vi "wykonajRuch.vi"(8 "error in (no error)":errorcluster, 9 "Wybór komory":T1, 10 "Akcja":T2=enum."Sprawdź", 11 "LINX Resource in":T3) -> (0 "error out":errorcluster, 3 "LINX Resource out":T3)   [LabVIEW 2014]
uses:
  <vilib>/MakerHub/LINX/Private/Type Defs/LINX Ref.ctl
  <vilib>/MakerHub/LINX/Private/Type Defs/Platform.ctl
  <vilib>/MakerHub/LINX/Private/Type Defs/Interface.ctl
  <vilib>/MakerHub/LINX/Private/Device/Type Defs/LINX Device Config.ctl
  <vilib>/MakerHub/LINX/Private/Device/Type Defs/TCP Config.ctl
  <vilib>/MakerHub/LINX/Private/Device/Type Defs/Channels.ctl
  wczytajDaneDoRuchuVIs/Akcje_wczytywania_danych_do_ruchu.ctl
  wykonajRuchVIs/parametryKomorVIs/Wybor_komory.ctl
  Akcja_kontrolki.ctl
  <vilib>/MakerHub/LINX/LMH-LINX.lvlib
  <vilib>/MakerHub/LINX/Private/Device/Device.lvlib
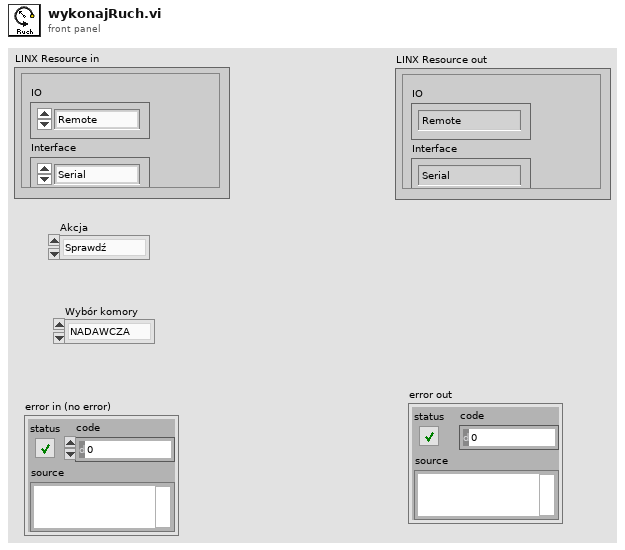
[diagram p1: front panel]
types:
  T1 = typedef "Wybor_komory.ctl" = enum16{"NADAWCZA", "ODBIORCZA"}
  T2 = typedef "Akcje_wczytywania_danych_do_ruchu.ctl" = enum16{"Init", "Reset ramienia", "Przygotuj listę", "Sprawdź", "Koniec"}
  T3 = typedef "LMH-LINX.lvlib/LINX Ref.ctl" = cluster{"IO":T4, "Interface":T5, "LINX Device Config":T6}
  T4 = typedef "LMH-LINX.lvlib/Platform.ctl" = enum16{"Remote", "Local"}
  T5 = typedef "LMH-LINX.lvlib/Interface.ctl" = enum16{"Serial", "TCP"}
  T6 = typedef "LMH-LINX.lvlib/Device.lvlib/LINX Device Config.ctl" = cluster{"Interface":T5, "COM Port":refnum<visa-resource-name>, "TCP Configuration":T7, "Device Family":u8, "Device ID":u8, "Device Name":string, "TCP Ref":refnum<k5>, "Channels":T8}
  T7 = typedef "LMH-LINX.lvlib/Device.lvlib/TCP Config.ctl" = cluster{"IP Address":string, "Port":u16}
  T8 = typedef "LMH-LINX.lvlib/Channels.ctl" = cluster{"DI":u8[], "DO":u8[], "AI":u8[], "AO":u8[], "PWM":u8[], "QE":u8[], "UART":u8[], "I2C 2":u8[], "SPI":u8[], "CAN":u8[], "Servo":u8[], "AI Ref (V)":dbl, "AI Resolution (Bits)":u8, "AO Ref (V)":dbl, "AO Resolution (Bits)":u8}
  T9 = typedef "Akcja_kontrolki.ctl" = enum16{"Czytaj", "Zapisz", "Reset"}
  T10 = typedef "Diody_zbior.ctl" = cluster{"Lewo":bool, "Prawo":bool, "Góra":bool, "Dół":bool, "Działanie":bool, "Czujnik":bool, "Pomiar":bool}
  T11 = typedef "RuchPoziomy.ctl" = enum16{"PRACA RĘCZNA", "COFAJ", "NAPRZÓD", "WYŁ."}
  T12 = typedef "RuchPionowy.ctl" = enum16{"WYŁ.", "GÓRA", "Dӣ", "PRACA RĘCZNA"}
  T13 = typedef "Przyciski_zbior.ctl" = cluster{"LEWO":bool, "PRAWO":bool, "GÓRA":bool, "Dӣ":bool, "Stop":bool, "Start":bool, "Praca ręczna":bool}
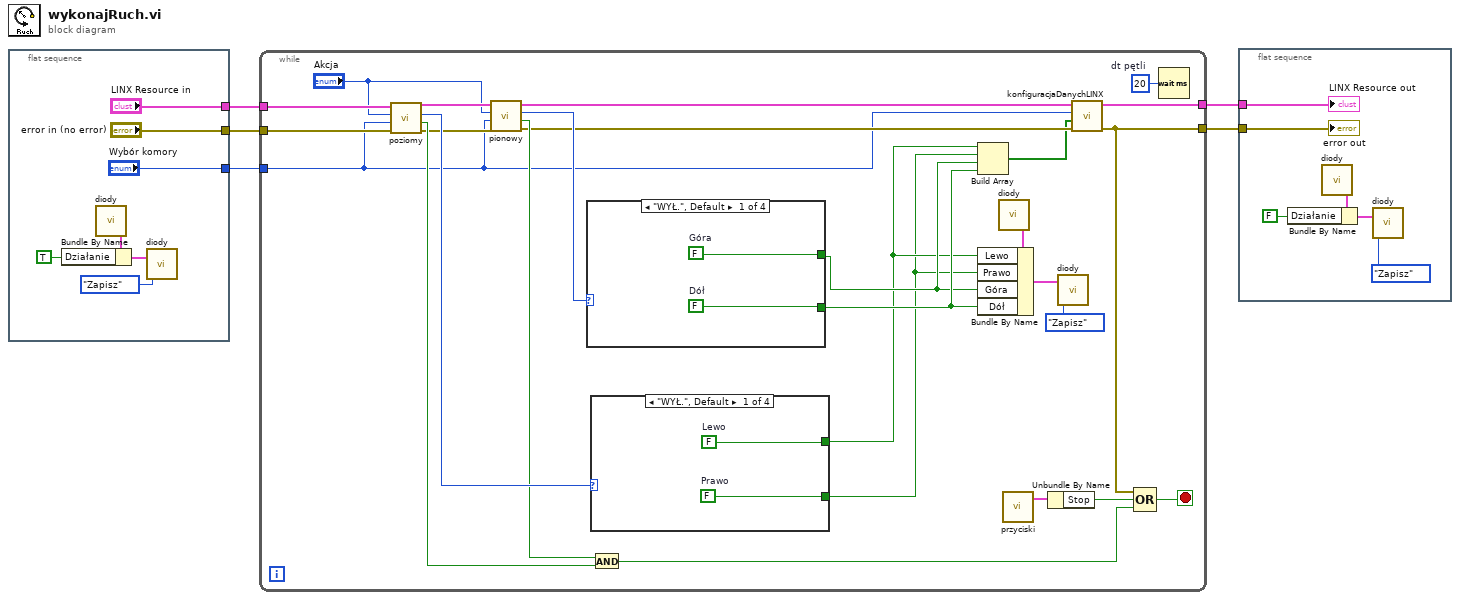
[diagram p0: block diagram]
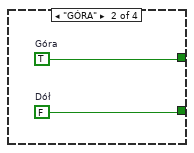
[diagram p2: hidden frame]
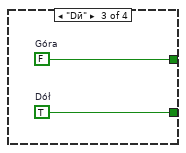
[diagram p3: hidden frame]
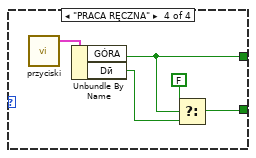
[diagram p4: hidden frame]
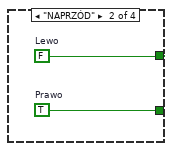
[diagram p5: hidden frame]
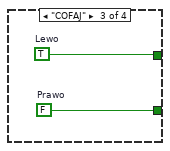
[diagram p6: hidden frame]
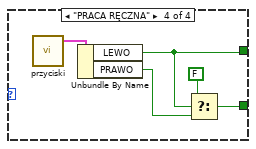
[diagram p7: hidden frame]
diagram:
  n1 = flat-sequence {
    tunnel: ["error in (no error)"] -> w5
    tunnel: ["LINX Resource in"] -> w4
    tunnel: ["Wybór komory"] -> w1
    frame #0 {
      n2 = call "diody.vi"() -> ("Wyjście"=w9:T10)  [unwired: 5 in]
      n3 = Bundle By Name(cluster=w9, "Działanie"=TRUE ("Wejście")) -> (w7:T10)
      n4 = call "diody.vi"("Akcja"=Akcja_kontrolki."Zapisz", "Wejście"=w7) -> ()  [unwired: 3 in, 1 out]
    }
  }
  n5 = while {
    tunnel: w4 -> [w31]
    tunnel: w5 -> [w34]
    tunnel: [w17] -> w2
    tunnel: [w16] -> w3
    tunnel: w1 -> [w13]
    stop <- w20 stop-if-true
    w39 = u32 20  # dt pętli
    n6 = call "poziomy.vi"("error in (no error)"=w34, "Wybór komory"=w13, "Akcja"="Akcja", "LINX Resource in"=w31) -> ("error out"=w19:errorcluster, "KONIEC"=w27:bool, "Aktualny stan"=w28:T11, "LINX Resource out"=w32:T3)  [unwired: 2 in]
    n7 = call "pionowy.vi"("error in"=w19, "Wybór komory"=w13, "Akcja"="Akcja", "LINX Resource in"=w32) -> ("error out"=w15:errorcluster, "KONIEC"=w26:bool, "Aktualny stan"=w29:T12, "LINX Resource out"=w18:T3)  [unwired: 2 in]
    n8 = case shown="\"WYŁ.\", Default" w29 {
      tunnel: [w41 w43 w45 w47] -> w25
      tunnel: [w40 w42 w44 w50] -> w33
      frame "WYŁ.", Default {
        w40 = FALSE  # Dół
        w41 = FALSE  # Góra
      }
      frame "GÓRA" {
        w42 = FALSE  # Dół
        w43 = TRUE  # Góra
      }
      frame "Dӣ" {
        w44 = TRUE  # Dół
        w45 = FALSE  # Góra
      }
      frame "PRACA RĘCZNA" {
        n9 = call "przyciski.vi"() -> ("Wyjście"=w48:T13)  [unwired: 5 in]
        n10 = Unbundle By Name(w48) -> ("GÓRA"=w47:bool, "Dӣ"=w46:bool)
        n11 = Select(t=FALSE, s=w47, f=w46) -> (s? t:f=w50:bool)
      }
    }
    n12 = case shown="\"WYŁ.\", Default" w28 {
      tunnel: [w52 w54 w56 w58] -> w24
      tunnel: [w51 w53 w55 w61] -> w23
      frame "WYŁ.", Default {
        w51 = FALSE  # Prawo
        w52 = FALSE  # Lewo
      }
      frame "NAPRZÓD" {
        w53 = TRUE  # Prawo
        w54 = FALSE  # Lewo
      }
      frame "COFAJ" {
        w55 = FALSE  # Prawo
        w56 = TRUE  # Lewo
      }
      frame "PRACA RĘCZNA" {
        n13 = call "przyciski.vi"() -> ("Wyjście"=w59:T13)  [unwired: 5 in]
        n14 = Unbundle By Name(w59) -> ("LEWO"=w58:bool, "PRAWO"=w57:bool)
        n15 = Select(t=FALSE, s=w58, f=w57) -> (s? t:f=w61:bool)
      }
    }
    n16 = And(x=w26, y=w27) -> (x .and. y?=w21:bool)
    n17 = Build Array(w24, w23, w25, w33) -> (w14:bool[])
    n18 = call "diody.vi"() -> ("Wyjście"=w36:T10)  [unwired: 5 in]
    n19 = Bundle By Name(cluster=w36, "Lewo"=w24, "Prawo"=w23, "Góra"=w25, "Dół"=w33) -> (w35:T10)
    n20 = call "przyciski.vi"() -> ("Wyjście"=w38:T13)  [unwired: 5 in]
    n21 = Unbundle By Name(w38) -> ("Stop"=w22:bool)
    n22 = call "diody.vi"("Akcja"=Akcja_kontrolki."Zapisz", "Wejście"=w35) -> ()  [unwired: 3 in, 1 out]
    n23 = call "konfiguracjaDanychLINX.vi"("Error In"=w15, "Kierunki"=w14, "Wybór komory"=w13, "LINX Resource"=w18) -> ("Error Out"=w16:errorcluster, "LINX Out"=w17:T3)  [unwired: 6 in]
    n24 = Compound Arithmetic op=OR(w16, w22, w21) -> (w20:bool)
    n25 = Wait (ms)(milliseconds to wait=w39) -> ()  [unwired: 1 out]
  }
  n26 = flat-sequence {
    tunnel: w3 -> [w67]
    tunnel: w2 -> [w66]
    frame #0 {
      n27 = call "diody.vi"() -> ("Wyjście"=w64:T10)  [unwired: 5 in]
      n28 = Bundle By Name(cluster=w64, "Działanie"=FALSE ("Wejście")) -> (w62:T10)
      n29 = call "diody.vi"("Akcja"=Akcja_kontrolki."Zapisz", "Wejście"=w62) -> ()  [unwired: 3 in, 1 out]
      "error out" <- w67
      "LINX Resource out" <- w66
    }
  }
